vi "Available AI.vi"(8 "error in (no error)":errorcluster, 11 "VisaComms in":refnum<class "VisaComms.lvclass">) -> (0 "error out":errorcluster, 2 "Available AI":T1[](array[typedef]), 3 "VisaComms out":refnum<class "VisaComms.lvclass">)   [LabVIEW 2024, in "CTI.lvlib" / "VisaComms.lvclass"]
uses:
  VisaComms.lvclass
  Available AI.ctl
  ADC Number.ctl
  GPIO Number.ctl
  VisaComms.lvclass/VisaComms.ctl
  Clean Visa Errors.vi
  CTI.lvlib
panel:
  out "Buffer":string
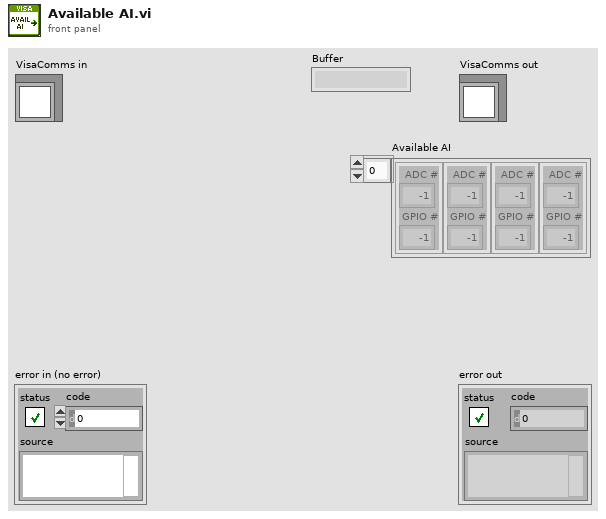
[diagram p1: front panel]
types:
  T1 = typedef "CTI.lvlib/Available AI.ctl" = cluster{"ADC #":T2, "GPIO #":T3}
  T2 = typedef "CTI.lvlib/ADC Number.ctl" = i8
  T3 = typedef "CTI.lvlib/GPIO Number.ctl" = i8
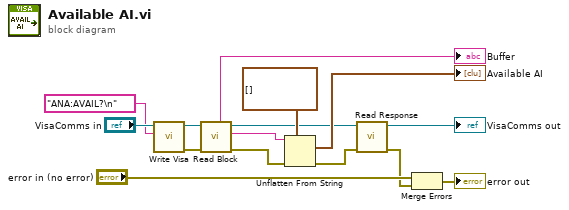
[diagram p0: block diagram]
diagram:
  n1 = call "Write Visa.vi"("write buffer"="ANA:AVAIL?\n", "VisaComms in"="VisaComms in") -> ("error out"=w11:errorcluster, "VisaComms out"=w12:refnum<class "VisaComms.lvclass">)  [unwired: 7 in, 1 out]
  n2 = call "Read Block.vi"("error in (no error)"=w11, "VisaComms in"=w12) -> ("error out"=w15:errorcluster, "Block"=w10:string, "VisaComms out"=w2:refnum<class "VisaComms.lvclass">, "Buffer"=→"Buffer":string)  [unwired: 6 in]
  n3 = Unflatten From String(type=T1[] [] ("Available AI"), binary string=w10, error in (no error)=w15) -> (value=→"Available AI":T1[], error out=w7:errorcluster)  [unwired: 2 in, 1 out]
  n4 = call "Read Response.vi"("error in (no error)"=w7, "VisaComms in"=w2) -> ("error out"=w3:errorcluster, "VisaComms out"=→"VisaComms out":refnum<class "VisaComms.lvclass">)  [unwired: 6 in, 2 out]
  n5 = Merge Errors("error in (no error)", w3) -> (→"error out":errorcluster)
